vi "valves_flushpath.vi"(0 "COM4 in":refnum<k24>, 2 "Input solution":dbl=1.0, 5 "error in":errorcluster) -> (6 "COM4 out":refnum<k24>, 8 "error out":errorcluster)   [LabVIEW 2018]
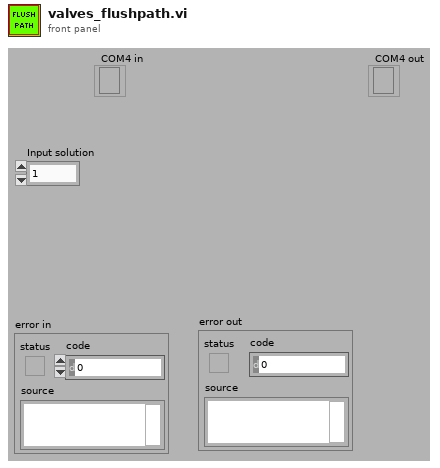
[diagram p1: front panel]
types:
  T1 = cluster{"Op A":u8[], "Op B":u8[], "Op C":u8[], "open":u8[], "L 3 A":u8[], "L 4 A 16":u8[], "F1 A":u8[], "L 4 A 34":u8[], "L 4 A 5":u8[], "FPw1 A":u8[], "L 2 A":u8[], "L 1 C FS":u8[], "L 2 C FS":u8[], "L 4 C 456 FS":u8[], "L 4 C 123 FS":u8[], "L 1 A":u8[], "L 1 C":u8[], "L 2 C":u8[], "L 4 C 456":u8[], "L 4 C 123":u8[], "FPw1 C":u8[], "F1 B":u8[], "F1 C":u8[], "F2 C":u8[], "F5 C":u8[]}
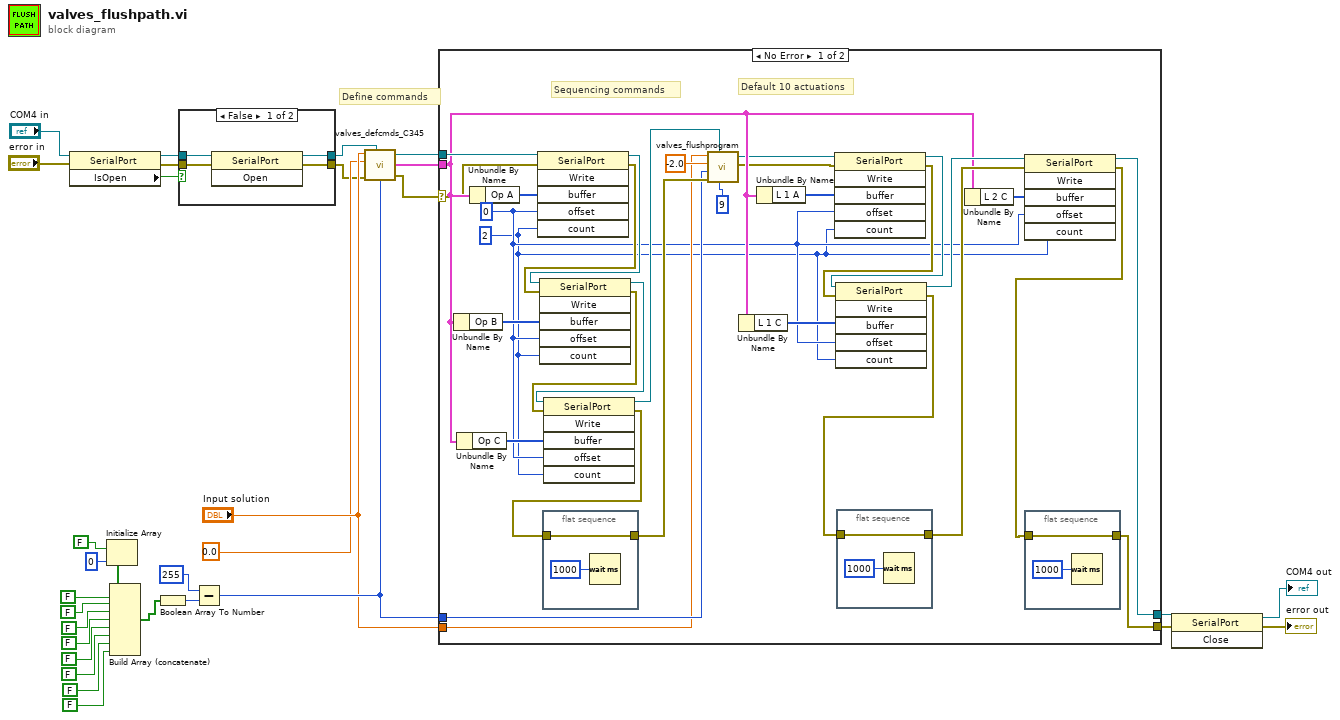
[diagram p0: block diagram]
diagram:
  # "Define commands"
  n1 = property class="SerialPort"(reference="COM4 in", error in="error in") -> (reference out=w9:refnum<k24>, error out=w10:errorcluster, "IsOpen"=w11:bool)
  n2 = Initialize Array(FALSE, 0 ("dimension size")) -> (w28:bool[])
  n3 = Build Array (concatenate)(w28, FALSE, FALSE, FALSE, FALSE, FALSE, FALSE, FALSE, FALSE) -> (w15:bool[])
  n4 = Boolean Array To Number(Boolean array=w15) -> (number=w17:u32)
  n5 = case shown="False" w11 {
    tunnel: [w32 w37] -> w8
    tunnel: [w33 w36] -> w7
    tunnel: w10 -> [w34 w36]
    tunnel: w9 -> [w35 w37]
    frame False {
      n6 = invoke class="SerialPort" method="Open"(reference=w35, error in=w34) -> (reference out=w32:refnum<k24>, error out=w33:errorcluster)  [unwired: 1 in, 1 out]
    }
    frame True {
    }
  }
  n7 = Subtract(x=u32 255, y=w17) -> (x-y=w14:u32)
  n8 = call "valves_defcmds_C345.vi"("Input solution"="Input solution", "Add to C"=0.0, "Rings to open"=w14, "error in"=w7, "COM4 in"=w8) -> ("COM4 out"=w29:refnum<k24>, "Commands out"=w30:T1, "error out"=w31:errorcluster)
  n9 = case shown="No Error" w31 {
    selector: w31 -> [w56 w77]
    tunnel: w29 -> [w69 w76]
    tunnel: [w47 w77] -> w3
    tunnel: w30 -> [w57 _]
    tunnel: w14 -> [w50 _]
    tunnel: "Input solution" -> [w48 _]
    tunnel: [w46 w76] -> w4
    frame No Error {
      w38 = 2 ("count")
      w39 = 0 ("offset")
      # "Default 10 actuations"
      # "Sequencing commands"
      n10 = Unbundle By Name(w57) -> ("Op B"=w44:u8[])
      n11 = Unbundle By Name(w57) -> ("Op C"=w43:u8[])
      n12 = Unbundle By Name(w57) -> ("Op A"=w45:u8[])
      n13 = invoke class="SerialPort" method="Write"(reference=w69, error in=w56, "buffer"=w45, "offset"=w39, "count"=w38) -> (reference out=w68:refnum<k24>, error out=w67:errorcluster)  [unwired: 1 in, 4 out]
      n14 = invoke class="SerialPort" method="Write"(reference=w68, error in=w67, "buffer"=w44, "offset"=w39, "count"=w38) -> (reference out=w66:refnum<k24>, error out=w65:errorcluster)  [unwired: 1 in, 4 out]
      n15 = flat-sequence {
        tunnel: [w74] -> w52
        tunnel: w64 -> [w74]
        frame #0 {
          n16 = Wait (ms)(milliseconds to wait=u32 1000) -> ()  [unwired: 1 out]
        }
      }
      n17 = invoke class="SerialPort" method="Write"(reference=w66, error in=w65, "buffer"=w43, "offset"=w39, "count"=w38) -> (reference out=w55:refnum<k24>, error out=w64:errorcluster)  [unwired: 1 in, 4 out]
      n18 = call "valves_flushprogram.vi"("Input solution"=w48, "COM4 in"=w55, "Add to C"=-2.0, "Rings to open"=w50, "Cycles"=9 ("Input solution"), "error in"=w52) -> ("COM4 out"=w54:refnum<k24>, "error out"=w53:errorcluster)  [unwired: 1 in]
      n19 = Unbundle By Name(w57) -> ("L 1 C"=w41:u8[])
      n20 = Unbundle By Name(w57) -> ("L 1 A"=w42:u8[])
      n21 = invoke class="SerialPort" method="Write"(reference=w54, error in=w53, "buffer"=w42, "offset"=w39, "count"=w38) -> (reference out=w61:refnum<k24>, error out=w63:errorcluster)  [unwired: 1 in, 4 out]
      n22 = invoke class="SerialPort" method="Write"(reference=w61, error in=w63, "buffer"=w41, "offset"=w39, "count"=w38) -> (reference out=w60:refnum<k24>, error out=w62:errorcluster)  [unwired: 1 in, 4 out]
      n23 = flat-sequence {
        tunnel: [w72] -> w59
        tunnel: w62 -> [w72]
        frame #0 {
          n24 = Wait (ms)(milliseconds to wait=u32 1000) -> ()  [unwired: 1 out]
        }
      }
      n25 = Unbundle By Name(w57) -> ("L 2 C"=w40:u8[])
      n26 = invoke class="SerialPort" method="Write"(reference=w60, error in=w59, "buffer"=w40, "offset"=w39, "count"=w38) -> (reference out=w46:refnum<k24>, error out=w58:errorcluster)  [unwired: 1 in, 4 out]
      n27 = flat-sequence {
        tunnel: [w70] -> w47
        tunnel: w58 -> [w70]
        frame #0 {
          n28 = Wait (ms)(milliseconds to wait=u32 1000) -> ()  [unwired: 1 out]
        }
      }
    }
    frame Error {
    }
  }
  n29 = invoke class="SerialPort" method="Close"(reference=w4, error in=w3) -> (reference out=→"COM4 out":refnum<k24>, error out=→"error out":errorcluster)  [unwired: 1 in, 1 out]
